vi "DEV testing Action Engine not wrapped.vi"() -> ()   [LabVIEW 2018, in "Database.lvlib"]
uses:
  Database.lvlib
  Action.ctl
panel:
  out "data":string[][](array[string])
  out "Query":string
  out "Query output":variant
  out "Cols and Col Info":variant
  out "Output":variant
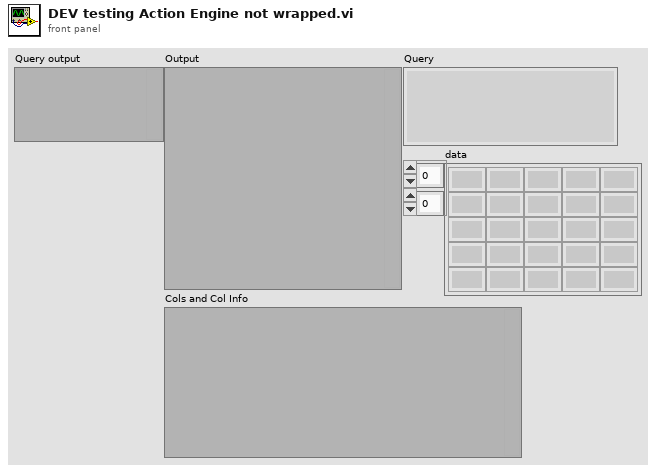
[diagram p1: front panel]
types:
  T1 = typedef "Database.lvlib/Action.ctl" = enum16{"Init", "List Tables", "List Columns", "Query", "Close"}
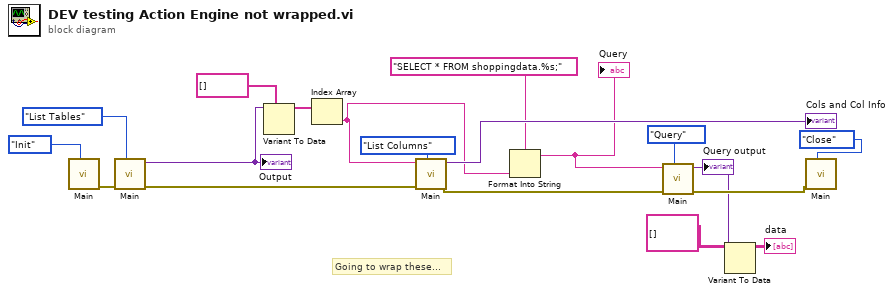
[diagram p0: block diagram]
diagram:
  # "Going to wrap these..."
  n1 = call "Main.vi"("Action"=Action."Init") -> ("Error Out"=w19:errorcluster)  [unwired: 9 in, 1 out]
  n2 = call "Main.vi"("Action"=Action."List Tables", "Error In"=w19) -> ("Error Out"=w15:errorcluster, "Output"=w13:variant)  [unwired: 8 in]
  "Output" <- w13
  n3 = Variant To Data(type=string[] [], Variant=w13) -> (data=w10:string[])  [unwired: 1 in, 1 out]
  n4 = Index Array(array=w10) -> (element=w8:string)  [unwired: 1 in]
  n5 = call "Main.vi"("Action"=Action."List Columns", "Error In"=w15, "Input"=w8) -> ("Error Out"=w5:errorcluster, "Output"=→"Cols and Col Info":variant)  [unwired: 7 in]
  n6 = Format Into String(format string="SELECT * FROM shoppingdata.%s;", w8) -> (resulting string=w7:string)  [unwired: 2 in, 1 out]
  "Query" <- w7
  n7 = call "Main.vi"("Action"=Action."Query", "Error In"=w5, "Input"=w7) -> ("Error Out"=w4:errorcluster, "Output"=w3:variant)  [unwired: 7 in]
  "Query output" <- w3
  n8 = Variant To Data(type=string[][] [], Variant=w3) -> (data=→"data":string[][])  [unwired: 1 in, 1 out]
  n9 = call "Main.vi"("Action"=Action."Close", "Error In"=w4) -> ()  [unwired: 8 in, 2 out]
